vi "Adquirir entre cursores.vi"(0 "WaveformGraph in":refnum<vi>, 1 "Input Cluster":T1, 2 "Flag":i32, 3 "Cursor 0":dbl, 4 "Cursor 1":dbl, 5 "error in":errorcluster) -> (15 "Output Cluster":T1, 19 "error out":errorcluster)   [LabVIEW 2020]
uses:
  TypeDef's/Dados consumidor.ctl
  <vilib>/Waveform/WDTOps.llb/WDT Get Waveform Subset DBL.vi
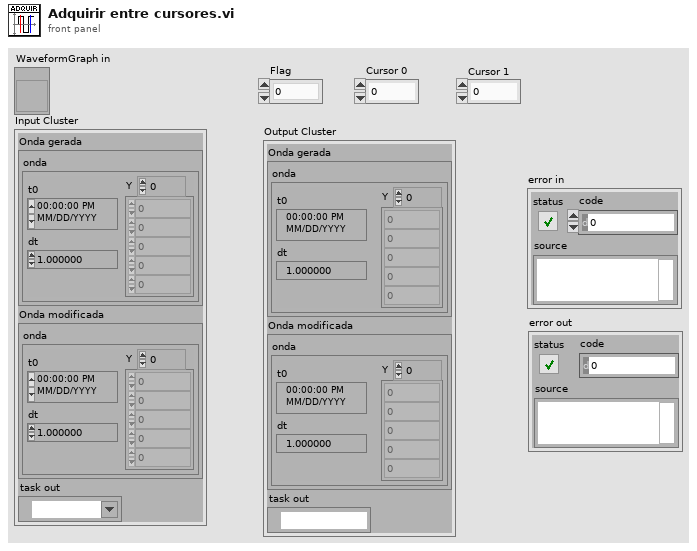
[diagram p1: front panel]
types:
  T1 = typedef "Dados consumidor.ctl" = cluster{"Onda gerada":cluster{"onda":waveform(dbl)}, "Onda modificada":cluster{"onda":waveform(dbl)}, "task out":refnum<k21>}
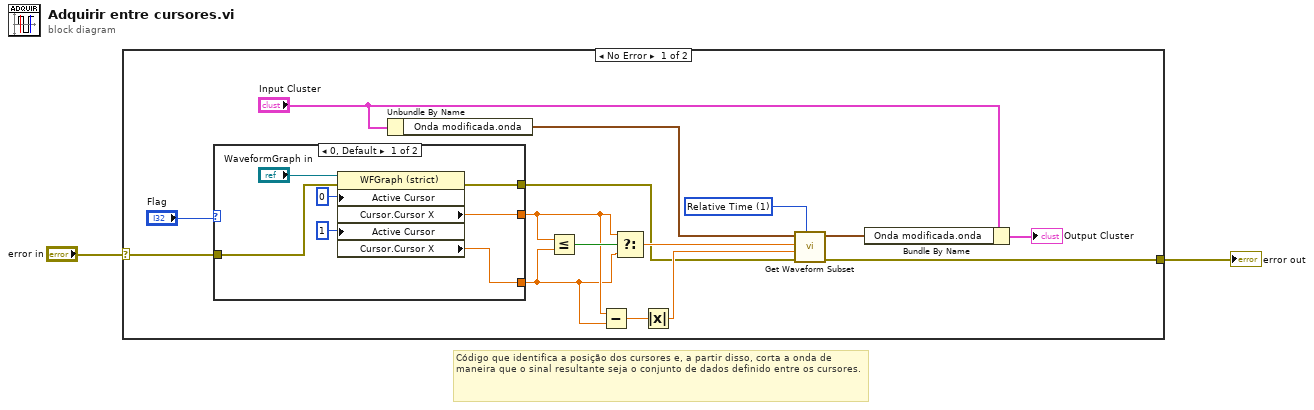
[diagram p0: block diagram]
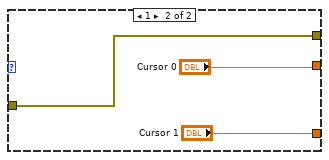
[diagram p2: hidden frame]
diagram:
  # "Código que identifica a posição dos cursores e, a partir disso, corta a onda de maneira que o sinal resultante seja o conjunto de dados definido entre os cursores."
  n1 = case shown="No Error" "error in" {
    selector: "error in" -> [w5 w28]
    tunnel: [w4 w28] -> w1
    frame No Error {
      w16 = u16 1 items=["Samples", "Relative Time"] ("start/duration format")
      n2 = case shown="0, Default" "Flag" {
        tunnel: [w21 "Cursor 0"] -> w10
        tunnel: [w20 "Cursor 1"] -> w9
        tunnel: [w19 w25] -> w7
        tunnel: w5 -> [w18 w25]
        frame 0, Default {
          n3 = property on="Property Node" class="WFGraph (strict)"(reference="WaveformGraph in", error in=w18, "Active Cursor"=u32 0, "Active Cursor"=u32 1) -> (error out=w19:errorcluster, "Cursor.Cursor X"=w21:dbl, "Cursor.Cursor X"=w20:dbl)  [unwired: 1 out]
        }
        frame 1 {
        }
      }
      n4 = Unbundle By Name("Input Cluster") -> ("Onda modificada.onda"=w15:waveform(dbl))
      n5 = Less Or Equal?(x=w10, y=w9) -> (x <= y?=w13:bool)
      n6 = Subtract(x=w10, y=w9) -> (x-y=w11:dbl)
      n7 = Select(t=w10, s=w13, f=w9) -> (s? t:f=w12:dbl)
      n8 = Absolute Value(x=w11) -> (abs(x)=w8:dbl)
      n9 = call-poly <vilib>:"Get Waveform Subset.vi"("start/duration format"=w16, "error in (no error)"=w7, "duration"=w8, "start samples/time"=w12, "waveform in"=w15) -> ("error out"=w4:errorcluster, "waveform out"=w6:waveform(dbl))  [unwired: 1 in, 2 out]
      n10 = Bundle By Name(cluster="Input Cluster", "Onda modificada.onda"=w6) -> (→"Output Cluster":T1)
    }
    frame Error {
    }
  }
  "error out" <- w1
